vi "Write Headers.vi"(1 "Channel Names":string[](array[string])=["Channel 1", "Channel 2"], 2 "Sampling Rates":string[](array[string])=["Channel 1", "Channel 2"], 3 "Description":string="Description goes here") -> (0 "Full Header String":string)   [LabVIEW 2015]
doc: "This is the file which compiles all of the header stuff and writes it to the text file <b> THIS IS NECESSARY FOR LVimport.m TO WORK </b>"
panel:
  out "Sampling Rate String":string
  out "Channel String":string
  out "current time":timestamp
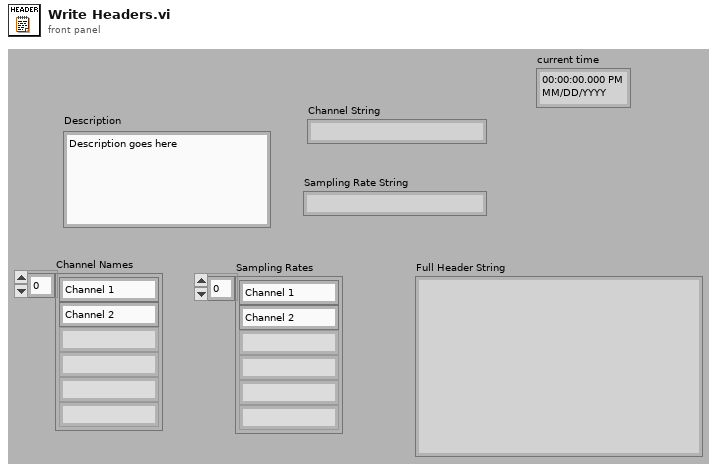
[diagram p1: front panel]
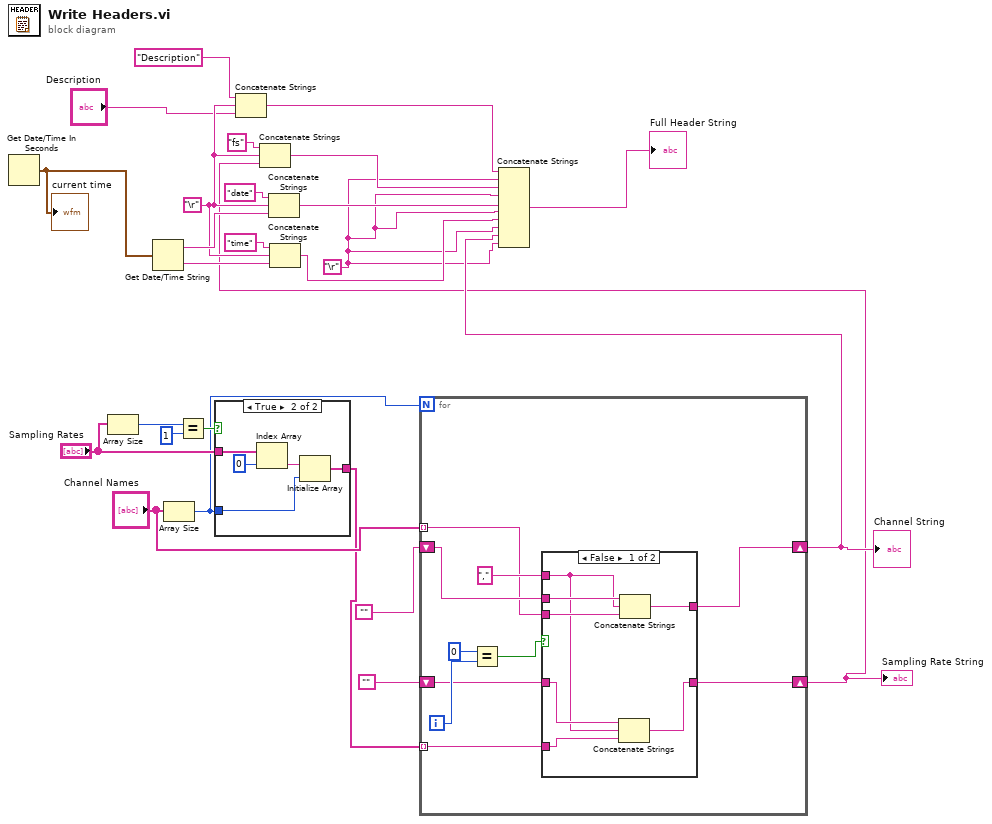
[diagram p0: block diagram]
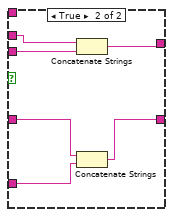
[diagram p3: hidden frame]
diagram:
  w20 = "\r"
  w10 = "\r"
  n1 = Get Date/Time In Seconds() -> (seconds since 1Jan1904=w26:timestamp)
  "current time" <- w26
  n2 = Array Size(array="Sampling Rates") -> (size(s)=w7:i32)
  n3 = Get Date/Time String(seconds (now)=w26) -> (date string=w23:string, time string=w22:string)  [unwired: 2 in]
  n4 = Array Size(array="Channel Names") -> (size(s)=w3:i32)
  n5 = Equal?(x=w7, y=1) -> (x = y?=w5:bool)
  n6 = case shown="True" w5 {
    tunnel: "Sampling Rates" -> [w27 w31]
    tunnel: w3 -> [_ w29]
    tunnel: [w27 w28] -> w2
    frame False {
    }
    frame True {
      n7 = Index Array(array=w31, index=0) -> (element=w32:string)
      n8 = Initialize Array(w32, w29) -> (w28:string[])
    }
  }
  n9 = Concatenate Strings("Description" ("string"), w20, "Description") -> (w15:string)
  n10 = Concatenate Strings("date", w20, w23) -> (w13:string)
  n11 = Concatenate Strings("time" ("string"), w20, w22) -> (w12:string)
  n12 = for {
    N: w3 -> [_]
    tunnel: "Channel Names" -> [w37] mode=indexing
    shift-right: [w36] -> w11
    shift-left: "" -> [w39]
    tunnel: w2 -> [w34] mode=indexing
    shift-right: [w33] -> w1
    shift-left: "" -> [w35]
    i -> [w42]
    n13 = Equal?(x=0, y=w42) -> (x = y?=w40:bool)
    n14 = case shown="False" w40 {
      tunnel: w39 -> [w46 w55]
      tunnel: "," -> [w43 _]
      tunnel: w37 -> [w49 w54]
      tunnel: [w48 w53] -> w36
      tunnel: w35 -> [w47 w52]
      tunnel: w34 -> [w45 w51]
      tunnel: [w44 w50] -> w33
      frame False {
        n15 = Concatenate Strings(w47, w43, w45) -> (w44:string)
        n16 = Concatenate Strings(w46, w43, w49) -> (w48:string)
      }
      frame True {
        n17 = Concatenate Strings(w55, w54) -> (w53:string)
        n18 = Concatenate Strings(w52, w51) -> (w50:string)
      }
    }
  }
  "Channel String" <- w11
  "Sampling Rate String" <- w1
  n19 = Concatenate Strings("fs", w20, w1) -> (w14:string)
  n20 = Concatenate Strings(w15, w10, w14, w10, w13, w10, w12, w10, w11, w10) -> (→"Full Header String":string)
